vi "mlink_scan_trigger_dio.vi"(7 "trigger type":T1, 8 "error in (no error)":errorcluster, 9 "dio":u8, 10 "level":u8, 11 "connection ID":i32=-1) -> (0 "error out":errorcluster, 3 "connection ID out":i32)   [LabVIEW 2009, in "MicroDAQ.lvlib" / "mlink.lvlib"]
doc: "This function configures DIO level trigger for AO/AI scan operation. The function shall be called after scan initialization function. The trigger argument determines if function affects AO or AI trigger settings. The dio argument defines digital input line number, level argument determines dio level on which acquisition or signal generation will be started."
uses:
  <instrlib>/MicroDAQ/Mlink library wraper/mlink.lvlib
  <instrlib>/MicroDAQ/Tools/Trigger type.ctl
  <instrlib>/MicroDAQ/MLink32.dll
  <instrlib>/MicroDAQ/MicroDAQ.lvlib
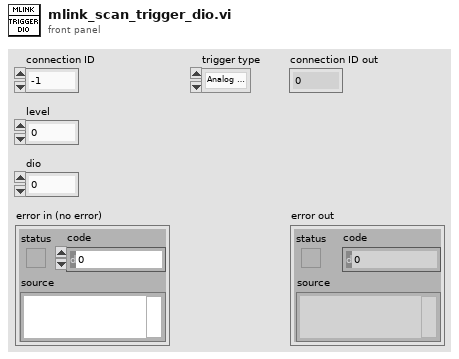
[diagram p1: front panel]
types:
  T1 = typedef "MicroDAQ.lvlib/Trigger type.ctl" = enum8{"Analog output", "Analog input"}
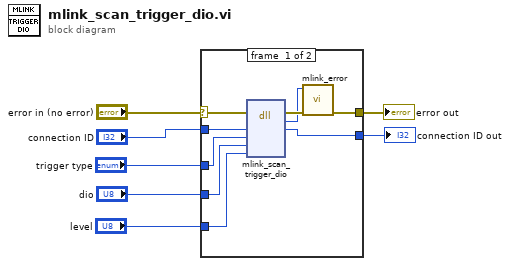
[diagram p0: block diagram]
diagram:
  n1 = case shown="No Error" "error in (no error)" {
    selector: "error in (no error)" -> [w16 w18]
    tunnel: "connection ID" -> [w15 w17]
    tunnel: [w14 w17] -> w5
    tunnel: [w11 w18] -> w4
    tunnel: "trigger type" -> [w10 _]
    tunnel: "dio" -> [w9 _]
    tunnel: "level" -> [w8 _]
    frame #0 {
      n2 = dll-call lib="C:/Program Files (x86)/National Instruments/LabVIEW 2009/instr.lib/MicroDAQ/MLink32.dll" fn="mlink_scan_trigger_dio" ("MLink64.dll:mlink_dsp_run")(error in=w16, "link_fd"=w15, "trigger"=w10, "dio"=w9, "level"=w8) -> (error out=w13:errorcluster, "return type"=w12:i32, "link_fd"=w14:i32)  [unwired: 5 in, 1 out]
      n3 = call <instrlib>:"mlink_error.vi"("error in (no error)"=w13, "error code"=w12) -> ("error out"=w11:errorcluster)  [unwired: 9 in]
    }
    frame #1 {
    }
  }
  "connection ID out" <- w5
  "error out" <- w4
